vi "Hit Splitter.vi"(8 "error in (no error)":errorcluster, 10 "Coords":T2, 11 "IObject in":refnum<class "IObject.lvclass">) -> (0 "error out":errorcluster, 1 "Hit?":bool, 2 "Limits":cluster{"Left":i16, "Right":i16}, 3 "IObject out":refnum<class "IObject.lvclass">, 4 "Slider":T1={"Left"=0.0, "Top"=0.0, "Right"=1.0, "Bottom"=0.0}, 5 "vertical?":bool, 6 "Position":i16)   [LabVIEW 2021, in "IObject.lvclass"]
uses:
  IObject.lvclass
  <vilib>/Utility/miscctls.llb/LVPoint32TypeDef.ctl
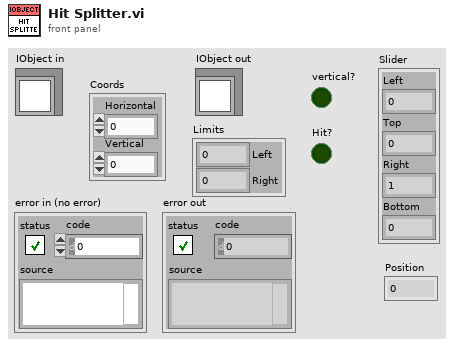
[diagram p1: front panel]
types:
  T1 = cluster{"Left":dbl, "Top":dbl, "Right":dbl, "Bottom":dbl}
  T2 = typedef "LVPoint32TypeDef.ctl" = cluster{"Horizontal":i32, "Vertical":i32}
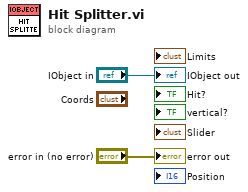
[diagram p0: block diagram]
diagram:
  "error out" <- "error in (no error)"
  "IObject out" <- "IObject in"
